vi "dfd_FXP PtByPt Even Symmetric FIR.vi"(6 "state in":i64[](array[numeric]), 7 "FXPOPs":T5[](array[typedef]) {"source" items=["Coef a/k"=0, "Coef b/v"=7, "Input"=1, "Output"=2, "Multiplicand"=3, "Product"=4, "Sum"=5, "Delay"=6, "Gain"=8]}, 8 "filtering statistics in":T4(array[cluster]) {"statistics information"."min value" format="%.2f"; "statistics information"."max value" format="%.2f"; "Quantizer Source" items=["Coefficients a/k"=0, "Coefficients b/v"=7, "Input"=1, "Output"=2, "Multiplicand"=3, "Product"=4, "Sum"=5, "Delay"=6]}, 10 "coef b (half stored)":i64[](array[numeric]), 11 "x":T7={"value"=0, "wl"=0, "iwl"=0, "Signed"=TRUE} {"value" format="%.0x"}) -> (0 "filtering statistics out":T4(array[cluster]) {"statistics information"."min value" format="%.2f"; "statistics information"."max value" format="%.2f"; "Quantizer Source" items=["Coefficients a/k"=0, "Coefficients b/v"=7, "Input"=1, "Output"=2, "Multiplicand"=3, "Product"=4, "Sum"=5, "Delay"=6]}, 3 "filtered x":T7={"value"=0, "wl"=0, "iwl"=0, "Signed"=TRUE} {"value" format="%.0x"}, 4 "state out":i64[](array[numeric]))   [LabVIEW 2017, in "NI_DigFilter_FXP.lvlib"]
uses:
  <vilib>/addons/Digital Filter Design/NI_DigFilter_FXP.lvlib
  <vilib>/addons/Digital Filter Design/_Objects.llb/dfd_DFXP Data Type (scaler).ctl
  <vilib>/addons/Digital Filter Design/_Objects.llb/dfd_DFXP Operation Parameter.ctl
  <vilib>/addons/Digital Filter Design/_Objects.llb/dfd_Internal Quantization Srcs.ctl
  <vilib>/addons/Digital Filter Design/_Objects.llb/DFD Quantization Sources.ctl
  <vilib>/addons/Digital Filter Design/_Objects.llb/DFD FXP Statistics Data.ctl
  <vilib>/addons/Digital Filter Design/_Objects.llb/dfd_DFXP Data Type (vector).ctl
  <vilib>/addons/Digital Filter Design/NI_DigFilterLicensed.lvlib
panel:
  in  "coef_b":T1
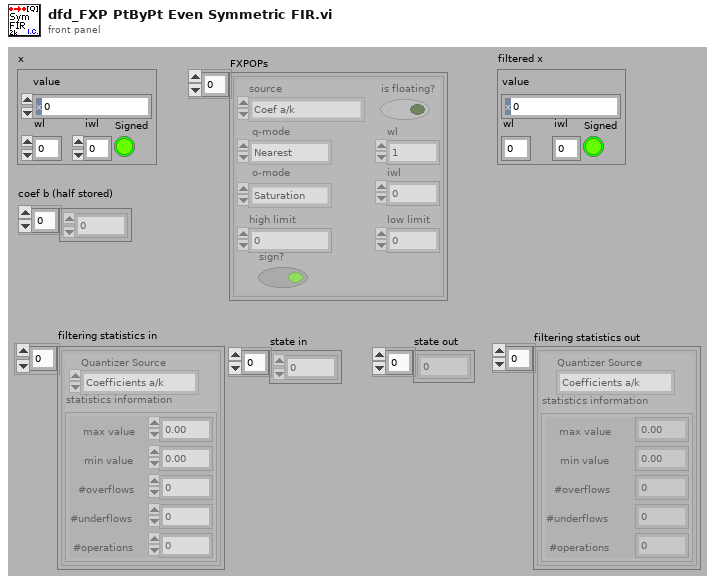
[diagram p1: front panel]
types:
  T1 = typedef "dfd_DFXP Data Type (vector).ctl" = cluster{"Values":i64[], "wl":i16, "iwl":i16}
  T2 = typedef "NI_DigFilterLicensed.lvlib/DFD Quantization Sources.ctl" = u16
  T3 = typedef "NI_DigFilterLicensed.lvlib/DFD FXP Statistics Data.ctl" = cluster{"max value":ext, "min value":ext, "#overflows":i32, "#underflows":i32, "#operations":i32}
  T4 = cluster{"Quantizer Source":T2, "statistics information":T3}[]
  T5 = typedef "dfd_DFXP Operation Parameter.ctl" = cluster{"source":T6, "is floating?":bool, "o-mode":enum16{"Saturation", "Wrap"}, "q-mode":enum16{"Nearest", "Truncation"}, "wl":i16, "high limit":i64, "low limit":i64, "iwl":i16, "sign?":bool}
  T6 = typedef "NI_DigFilterLicensed.lvlib/dfd_Internal Quantization Srcs.ctl" = u16
  T7 = typedef "dfd_DFXP Data Type (scaler).ctl" = cluster{"value":i64, "wl":i16, "iwl":i16, "Signed":bool}
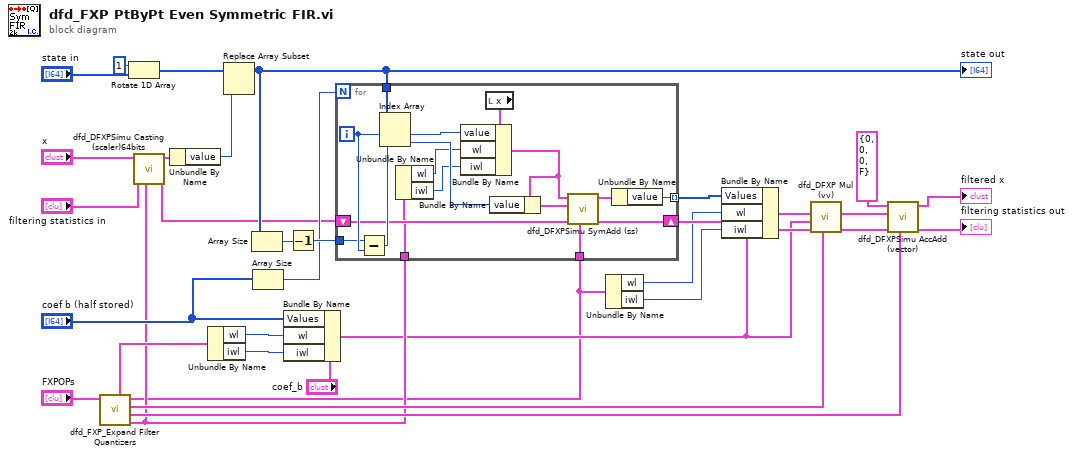
[diagram p0: block diagram]
diagram:
  n1 = call <vilib>:"dfd_FXP_Expand Filter Quantizers.vi"("FXPOPs"="FXPOPs") -> ("Delay"=w6:T5, "Sum"=w21:T5, "Product"=w20:T5, "Multiplicand"=w3:T5, "Coefficient b/v"=w10:T5)  [unwired: 6 out]
  n2 = Rotate 1D Array(1:"state in", 2:1 ("n")) -> (0:w33:i64[])
  n3 = call <vilib>:"dfd_DFXPSimu Casting (scaler)64bits.vi"("op params"=w6, "filtering statistics in"="filtering statistics in", "Value in"="x") -> ("filtering statistics out"=w16:T4, "Value out"=w30:T7)  [unwired: 2 in, 5 out]
  n4 = Unbundle By Name(w30) -> ("value"=w7:i64)
  n5 = Unbundle By Name(w10) -> ("wl"=w9:i16, "iwl"=w8:i16)
  n6 = Replace Array Subset(array=w33, new element=w7) -> (w18:i64[])  [unwired: 1 in]
  "state out" <- w18
  n7 = Array Size(array=w18) -> (size(s)=w28:i32)
  n8 = Array Size(array="coef b (half stored)") -> (size(s)=w17:i32)
  n9 = Bundle By Name(cluster="coef_b", "Values"="coef b (half stored)", "wl"=w9, "iwl"=w8) -> (w4:T1)
  n10 = Decrement(x=w28) -> (x-1=w26:i32)
  n11 = for {
    N: w17 -> [_]
    tunnel: w18 -> [w50]
    tunnel: w26 -> [w47]
    tunnel: w3 -> [w44]
    shift-right: [w42] -> w15
    shift-left: w16 -> [w43]
    tunnel: [w34] -> w12 mode=indexing
    tunnel: w6 -> [w39]
    i -> [w49]
    n12 = Subtract(x=w47, y=w49) -> (x-y=w48:i32)
    n13 = Index Array(array=w50, index #1=w49, index #2=w48) -> (element #1=w46:i64, element #2=w45:i64)
    n14 = Unbundle By Name(w39) -> ("wl"=w38:i16, "iwl"=w37:i16)
    n15 = local read "x"() -> (w40:T7)
    n16 = Bundle By Name(cluster=w40, "value"=w46, "wl"=w38, "iwl"=w37) -> (w35:T7)
    n17 = Bundle By Name(cluster=w35, "value"=w45) -> (w36:T7)
    n18 = call <vilib>:"dfd_DFXPSimu SymAdd (ss).vi"("op params"=w44, "filtering statistics in"=w43, "value in 2"=w36, "value in 1"=w35) -> ("filtering statistics out"=w42:T4, "value out"=w41:T7)  [unwired: 2 in, 4 out]
    n19 = Unbundle By Name(w41) -> ("value"=w34:i64)
  }
  n20 = Unbundle By Name(w3) -> ("wl"=w2:i16, "iwl"=w1:i16)
  n21 = Bundle By Name(cluster=w4, "Values"=w12, "wl"=w2, "iwl"=w1) -> (w5:T1)
  n22 = call <vilib>:"dfd_DFXP Mul (vv).vi"("op params"=w20, "filtering statistics in"=w15, "Value in 2"=w4, "Value in"=w5) -> ("filtering statistics out"=w22:T4, "Value out"=w23:T1)  [unwired: 6 out]
  n23 = call <vilib>:"dfd_DFXPSimu AccAdd (vector).vi"("op params"=w21, "filtering statistics in"=w22, "addends"=w23, "acc in"=T7 {"value"=0, "wl"=0, "iwl"=0, "Signed"=FALSE}) -> ("filtering statistics out"=→"filtering statistics out":T4, "acc out"=→"filtered x":T7)  [unwired: 1 in, 5 out]
